vi "LVClass_ClosedLoopSmoothing Read ClosedLoopSmooth.vi"(8 "error in (no error)":errorcluster, 11 "ClosedLoopSmoothing in":refnum<class "ClosedLoopSmoothing.lvclass">) -> (0 "error out":errorcluster, 2 "ClosedLoopSmooth":i32, 3 "ClosedLoopSmoothing out":refnum<class "ClosedLoopSmoothing.lvclass">)   [LabVIEW 2020, in "ClosedLoopSmoothing.lvclass"]
uses:
  ClosedLoopSmoothing.lvclass
  ClosedLoopSmoothing.lvclass/ClosedLoopSmoothing.ctl
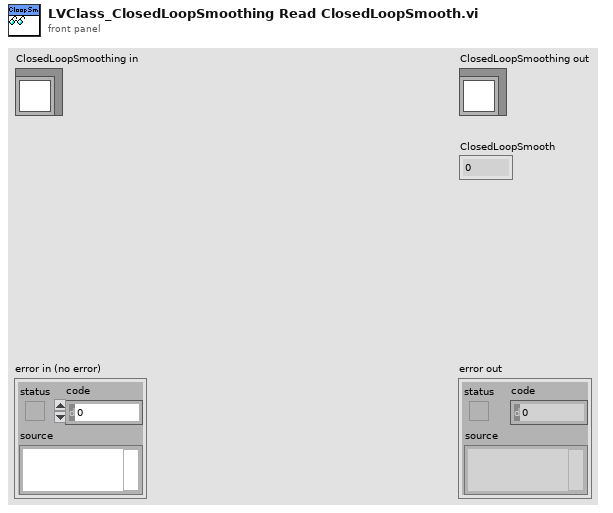
[diagram p1: front panel]
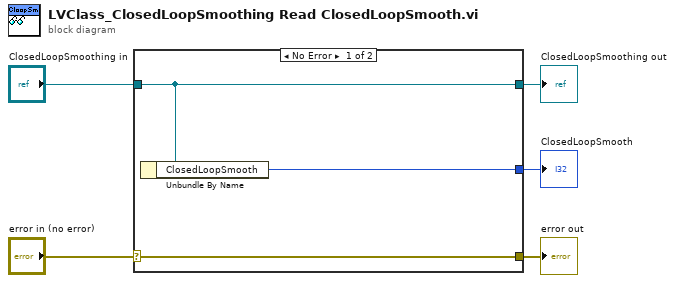
[diagram p0: block diagram]
diagram:
  n1 = case shown="No Error" "error in (no error)" {
    selector: "error in (no error)" -> [w8 w9]
    tunnel: [w8 w9] -> w4
    tunnel: [w7 w10] -> w2
    tunnel: "ClosedLoopSmoothing in" -> [w7 w10]
    tunnel: [w6 _] -> w1
    frame No Error {
      n2 = Unbundle By Name(w7) -> ("ClosedLoopSmooth"=w6:i32)
    }
    frame Error {
    }
  }
  "error out" <- w4
  "ClosedLoopSmoothing out" <- w2
  "ClosedLoopSmooth" <- w1
